vi "xyz-ast_localisation.vi"(4 "Positive angle":dbl, 5 "Gy":dbl[][](array[numeric]), 6 "Gthr":dbl[][](array[numeric]), 7 "Gx":dbl[][](array[numeric]), 8 "R":dbl, 9 "weights":dbl[](array[numeric]), 10 "B points":dbl[][](array[numeric])=[[5.0, 3.0], [6.0, 6.0]], 11 "A points":dbl[][](array[numeric])=[[0.0, 1.0], [2.0, 3.0]]) -> (2 "dR":dbl[](array[numeric]), 3 "XYZ":dbl[](array[numeric]))   [LabVIEW 2015]
doc: "INPUT\nR - radius of the window (should be >0.5)\nGx,Gy - horizontal and vertical local gradient images\nGthr - thresholded magnitude of local gradients (if not wired will be calculated from Gx,Gy)\nA points - 2xN array of first points that define lines\nB points - 2xN array of second points that define lines\nw - weights (1D array)\nPositive angle - angle in degrees that defines orientation of the image of the particle which corresponds to positive z-value\n\nOUTPUT\nXYZ - x,y position of the particle in pixels (for original image), z-value\ndR - distance from the center to each line (1D vector)\n\nThis vi calculates XYZ position of the fluorescent particle in astigmatism based microscopy. XY is found as a least square intersection point of gradient lines. The image of local gradients (Gthr) is splitted into 4 parts: TOP, LEFT, BOTTOM, RIGHT, relative to the particle center (cx,cy). The least-square intersection of all gradient lines (Gx, Gy) is calculated for each part. These centers are forming two lines: TOP-BOTTOM and LEFT-RIGHT, which are called axes (similar to ellipses axes). The major of two axes represents the magnitude of the z-value. The sign of the z-value is determined according to the angPos value which should correspond to the position of the long axis of the elliptical image of the particle. angPos is not required to be accurate, however, setting it to ~45 degrees off the real angle will create sporadic change in the sign and, therefore, in z-value.\n\nAuthor: Anatolii Kashchuk"
panel:
  out "center":dbl[][](array[numeric])
  # "This vi finds centroid and z-value from the image of a particle in astigmatism based microscopy\n\nAuthor: Anatolii Kashchuk"
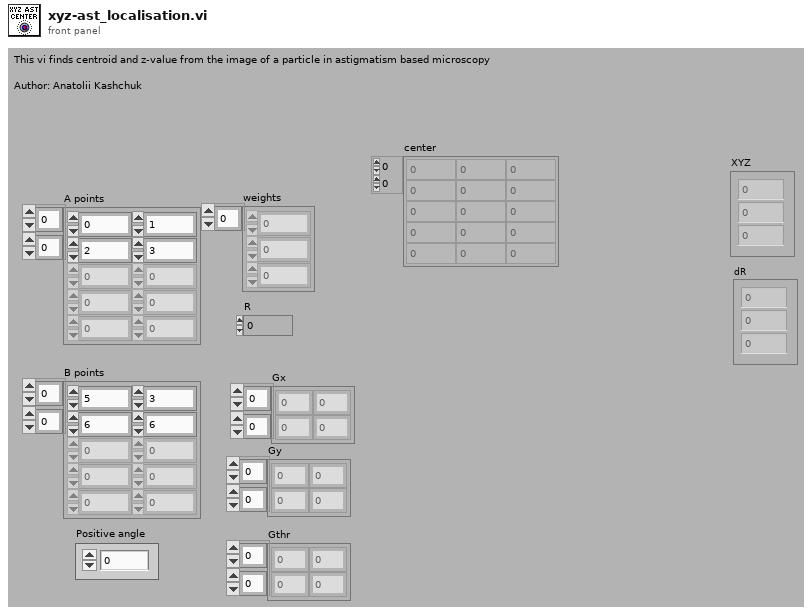
[diagram p1: front panel]
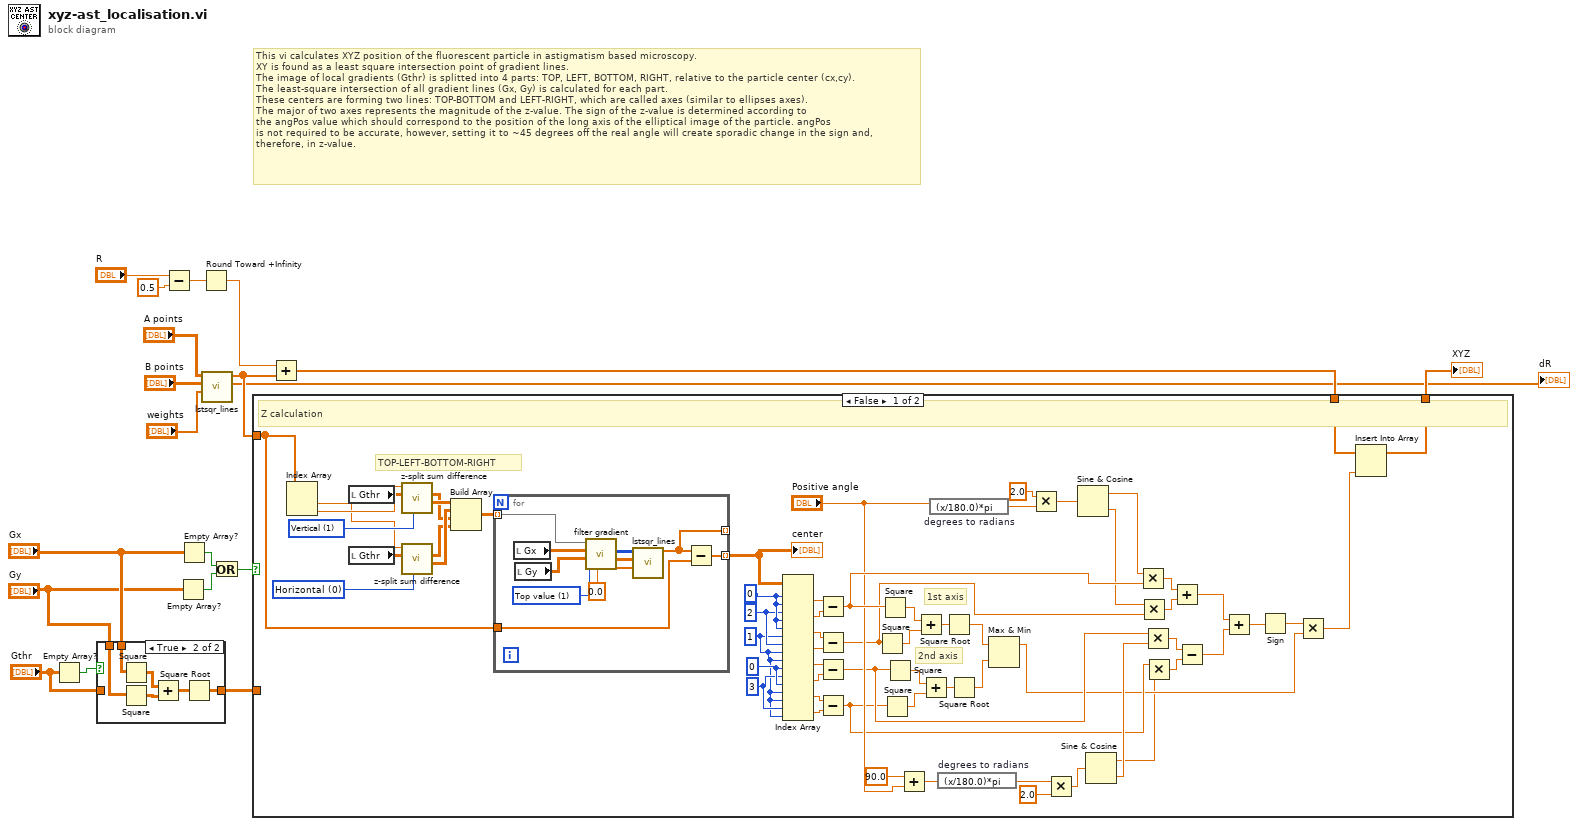
[diagram p0: block diagram]
diagram:
  # "This vi calculates XYZ position of the fluorescent particle in astigmatism based microscopy. \nXY is found as a least square intersection point of gradient lines. \nThe image of local gradients (Gthr) is splitted into 4 parts: TOP, LEFT, BOTTOM, RIGHT, relative to the particle center (cx,cy). \nThe least-square intersection of all gradient lines (Gx, Gy) is calculated for each part. \nThese centers are forming two lines: TOP-BOTTOM and LEFT-RIGHT, which are called axes (similar to ellipses axes). \nThe major of two axes represents the magnitude of the z-value. The sign of the z-value is determined according to \nthe angPos value which should correspond to the position of the long axis of the elliptical image of the particle. angPos\nis not required to be accurate, however, setting it to ~45 degrees off the real angle will create sporadic change in the sign and, \ntherefore, in z-value."
  n1 = Empty Array?(array="Gthr") -> (empty?=w7:bool)
  n2 = case shown="True" w7 {
    tunnel: "Gx" -> [_ w23]
    tunnel: "Gy" -> [_ w22]
    tunnel: [w20 w21] -> w4
    tunnel: "Gthr" -> [w20 _]
    frame False {
    }
    frame True {
      n3 = Square(x=w23) -> (x^2=w25:dbl[][])
      n4 = Square(x=w22) -> (x^2=w24:dbl[][])
      n5 = Add(x=w25, y=w24) -> (x+y=w26:dbl[][])
      n6 = Square Root(x=w26) -> (sqrt(x)=w21:dbl[][])
    }
  }
  n7 = Subtract(x="R", y=0.5) -> (x-y=w14:dbl)
  n8 = Empty Array?(array="Gy") -> (empty?=w8:bool)
  n9 = Empty Array?(array="Gx") -> (empty?=w9:bool)
  n10 = Round Toward +Infinity(x=w14) -> (ceil(x): smallest int >= x=w15:dbl)
  n11 = call "lstsqr_lines.vi"("weights"="weights", "B points"="B points", "A points"="A points") -> ("dR"=→"dR":dbl[], "center"=w12:dbl[])  [unwired: 6 in, 1 out]
  n12 = Or(x=w9, y=w8) -> (x .or. y?=w2:bool)
  n13 = Add(x=w15, y=w12) -> (x+y=w11:dbl[])
  n14 = case shown="False" w2 {
    tunnel: w12 -> [w56 _]
    tunnel: w11 -> [w88 w101]
    tunnel: [w89 w101] -> w10
    tunnel: w4 -> [_ _]
    frame False {
      w65 = 3 ("disabled index (col)")
      w64 = 1 ("disabled index (col)")
      w72 = 2 ("index (row)")
      w66 = 0 ("disabled index (col)")
      w73 = 0 ("index (row)")
      w85 = u16 0 items=["Horizontal", "Vertical"] ("Text Ring")
      w87 = u16 1 items=["Horizontal", "Vertical"] ("Text Ring")
      # "2nd axis"
      # "X1\nX3\nY1\nY3\nX2\nX4\nY2\nY4"
      # "1st axis"
      # "TOP-LEFT-BOTTOM-RIGHT"
      # "Z calculation"
      n15 = Index Array(array=w56) -> (element #1=w84:dbl, element #2=w86:dbl)  [unwired: 2 in]
      n16 = local read "Gthr"() -> (w82:dbl[][])
      n17 = local read "Gthr"() -> (w83:dbl[][])
      n18 = call "z-split sum difference.vi"("split type"=w87, "G input"=w82, "center"=w86) -> ("left/top"=w81:dbl[][], "right/bottom"=w79:dbl[][])  [unwired: 6 in, 1 out]
      n19 = call "z-split sum difference.vi"("split type"=w85, "G input"=w83, "center"=w84) -> ("left/top"=w80:dbl[][], "right/bottom"=w78:dbl[][])  [unwired: 6 in, 1 out]
      n20 = Build Array(w81, w80, w79, w78) -> (w77:dbl[][][])
      n21 = for {
        tunnel: w77 -> [w100] mode=indexing
        tunnel: [w92] -> w76 mode=indexing
        tunnel: w56 -> [w91]
        tunnel: [w90] -> _ mode=indexing
        w96 = u16 1 items=["Top fraction", "Top value"] ("Threshold type")
        n22 = local read "Gx"() -> (w99:dbl[][])
        n23 = local read "Gy"() -> (w98:dbl[][])
        n24 = call "filter gradient.vi"("Threshold"=0.0, "Threshold type"=w96, "Gy"=w98, "Gx"=w99, "G"=w100) -> ("Weights"=w93:dbl[], "gradients"=w94:dbl[][], "centers"=w95:i32[][])  [unwired: 1 in, 3 out]
        n25 = call "lstsqr_lines.vi"("weights"=w93, "B points"=w94, "A points"=w95) -> ("center"=w90:dbl[])  [unwired: 6 in, 2 out]
        n26 = Subtract(x=w90, y=w91) -> (x-y=w92:dbl[])
      }
      "center" <- w76
      n27 = Index Array(array=w76, index (row) #1=w73, index (col) #1=w73, index (row) #2=w72, index (col) #2=w73, index (row) #3=w73, index (col) #3=w64, index (row) #4=w72, index (col) #4=w64, index (row) #5=w64, index (col) #5=w66, index (row) #6=w65, index (col) #6=w66, index (row) #7=w64, index (col) #7=w64, index (row) #8=w65, index (col) #8=w64) -> (element #1=w74:dbl, element #2=w75:dbl, element #3=w71:dbl, element #4=w70:dbl, element #5=w60:dbl, element #6=w59:dbl, element #7=w58:dbl, element #8=w57:dbl)
      n28 = Subtract(x=w74, y=w75) -> (x-y=w52:dbl)
      n29 = Subtract(x=w71, y=w70) -> (x-y=w43:dbl)
      n30 = Subtract(x=w60, y=w59) -> (x-y=w36:dbl)
      n31 = Subtract(x=w58, y=w57) -> (x-y=w34:dbl)
      n32 = Square(x=w43) -> (x^2=w68:dbl)
      n33 = Square(x=w52) -> (x^2=w69:dbl)
      n34 = Square(x=w34) -> (x^2=w62:dbl)
      n35 = Square(x=w36) -> (x^2=w61:dbl)
      n36 = Add(x=90.0, y="Positive angle") -> (x+y=w49:dbl)
      n37 = Add(x=w69, y=w68) -> (x+y=w67:dbl)
      n38 = Add(x=w61, y=w62) -> (x+y=w63:dbl)
      n39 = expression code="(x/180.0)*pi" "degrees to radians"("Positive angle") -> (w53:dbl)
      n40 = expression code="(x/180.0)*pi" "degrees to radians"(w49) -> (w47:dbl)
      n41 = Square Root(x=w67) -> (sqrt(x)=w55:dbl)
      n42 = Square Root(x=w63) -> (sqrt(x)=w54:dbl)
      n43 = Max & Min(x=w55, y=w54) -> (max(x,y)=w29:dbl)  [unwired: 1 out]
      n44 = Multiply(x=2.0 ("y"), y=w53) -> (x*y=w48:dbl)
      n45 = Multiply(x=w47, y=2.0) -> (x*y=w45:dbl)
      n46 = Sine & Cosine(0:w48) -> (1:w44:dbl, 2:w42:dbl)
      n47 = Sine & Cosine(0:w45) -> (1:w27:dbl, 2:w35:dbl)
      n48 = Multiply(x=w44, y=w52) -> (x*y=w41:dbl)
      n49 = Multiply(x=w42, y=w43) -> (x*y=w40:dbl)
      n50 = Multiply(x=w36, y=w35) -> (x*y=w38:dbl)
      n51 = Multiply(x=w34, y=w27) -> (x*y=w39:dbl)
      n52 = Add(x=w41, y=w40) -> (x+y=w33:dbl)
      n53 = Subtract(x=w38, y=w39) -> (x-y=w32:dbl)
      n54 = Add(x=w33, y=w32) -> (x+y=w31:dbl)
      n55 = Sign(1:w31) -> (0:w30:dbl)
      n56 = Multiply(x=w30, y=w29) -> (x*y=w28:dbl)
      n57 = Insert Into Array(array=w88, new element=w28) -> (w89:dbl[])  [unwired: 1 in]
    }
    frame True {
    }
  }
  "XYZ" <- w10
